vi "FUG_PowerSupply.SetOnOff.vi"(0 "i ref in":refnum<vi>, 2 "value":bool, 5 "error in (no error)":errorcluster, 7 "channelIndex":i32) -> (14 "i ref out":refnum<vi>, 19 "error out (no error)":errorcluster)   [LabVIEW 2014, in "FUG_PowerSupply.lvlib"]
doc: "This VI calculates the right current from the DB values, saves the actual set current to the I-Attribute and set´s the Set Current-Service."
uses:
  FUG_PowerSupply.lvlib
  CSCore/CSSystem/CoreDefs/CoreDefs.error_type.ctl
  CSCore/CSSystem/CoreDefs/CoreDefs.error_severity.ctl
  CSCore/CSApplicationBaseClasses/PSChannelBase/PSChannelBase.serviceType.ctl
  CSlibraries/UtilityLib/UtilityLib.valueStatus.ctl
  CSCore/CSApplicationBaseClasses/PSChannelBase/PSChannelBase.directionType.ctl
  CSlibraries-extern/DimLVEvent/LVDimInterface/LVDimInterface.lvlib
  CSCore/CSApplicationBaseClasses/PSChannelBase/PSChannelBase.lvlib
  CSlibraries/UtilityLib/UtilityLib.lvlib
  CSCore/CSSystem/CoreLib/CoreLib.lvlib
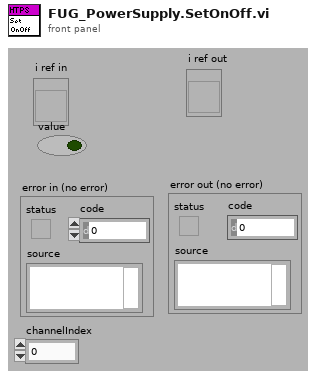
[diagram p1: front panel]
types:
  T1 = typedef "CoreDefs.error_severity.ctl" = enum16{"undefined", "information", "warning", "error", "fatal"}
  T2 = typedef "CoreDefs.error_type.ctl" = enum16{"no error", "can't load process", "can't unload process", "process does not exist", "can't install process", "can't remove process", "unknown function", "time out", "can't execute function", "duplicate queue name", "super not found", "caller queue invalid", "can't ping process", "unknown error", "VISA Error", "VISA timeout", "GPIB timeout", "GPIB error", "communication error", "data type mismatch", "can't read data from OPC server", "can't write data to OPC server", "OET error", "function not implemented", "process already exists", "invalid Shared Variable name", "error writing Shared Variable", "error reading Shared Variable", "invalid client name", "corrupt database", "unknown class", "call not authorized", "parameter out of range", "OET timeout: can't get data to modify", "invalid queue name", "requested operation incompatible with current state", "event undefined", "event disabled", "state undefined", "caller is not a friend", "EventBuilder: bad eventID", "EventBuilder: no DAQ devices", "a thread must not stop itself", "UNUSED ELEMENT4", "DiscArchiver: eventData incomplete", "DiscArchiver: eventData does not belong to run", "DiscArchiver: can't open file", "DiscArchiver: can't write to file", "DiscArchiver: available disc space low", "can't acquire semaphore", "error reading data from database", "notifier object is not existing", "can't register process", "can't unregister process", "illegal event type", "object disabled", "object already exists", "can't change state", "Instrument not found", "no connection to remote node", "invalid reference", "N/A", "UNUSED ELEMENT 1", "element not found", "illegal TCP/IP connection detected", "object does not exist", "invalid access ID", "unknown CS system", "invalid privilige", "unsupported data type", "unsupported server type", "IO server already exists", "Shared Variable already exists"}
  T3 = typedef "UtilityLib.lvlib/UtilityLib.valueStatus.ctl" = enum16{"no info available", "stand by/off", "on", "warning", "alarm/malfunction", "not implemented", "user action required", "important information", "system default", "control default", "indicator default", "button default"}
  T4 = typedef "PSChannelBase.lvlib/PSChannelBase.serviceType.ctl" = enum16{"onOff", "voltage", "current", "tripCurrent", "rampUpSpeed", "rampDownSpeed", "status"}
  T5 = typedef "PSChannelBase.lvlib/PSChannelBase.directionType.ctl" = enum16{"unknown", "update actual value", "update nominal value", "update both"}
  T6 = typedef "FUG_PowerSupply.lvlib/FUG_PowerSupply.i attribute.ctl" = cluster{"Type":string, "Elektrode Name":string, "CALC_FACTOR_SET_VOLTAGE":dbl, "CALC_FACTOR_GET_VOLTAGE":dbl, "CALC_FACTOR_GET_CURRENT":dbl, "CALC_FACTOR_SET_CURRENT ":dbl, "REG_VALUE":dbl, "Sign":bool, "setVoltID":i32, "setCurrentID":i32, "setPowerOnID":i32, "MaxVoltage":dbl}
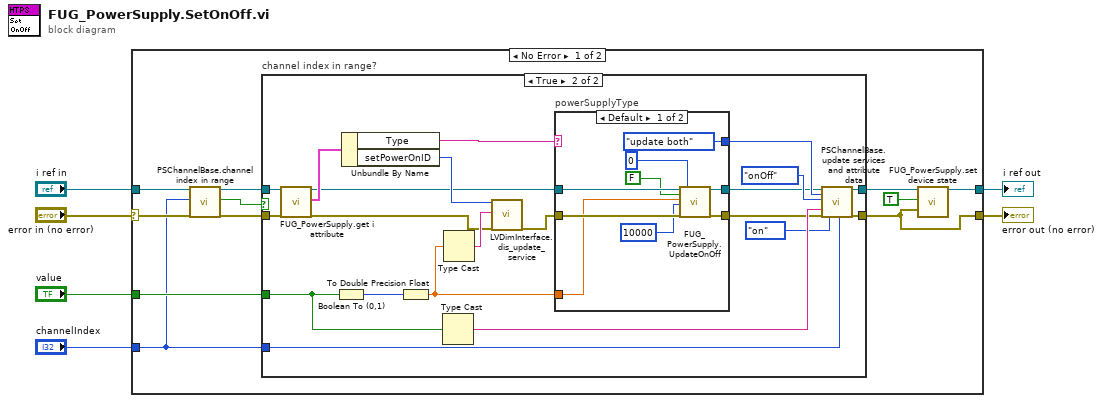
[diagram p0: block diagram]
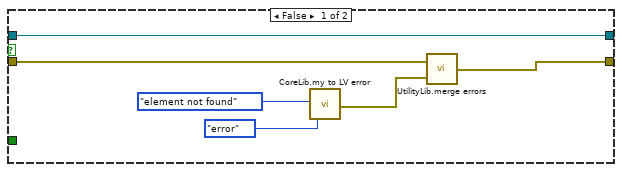
[diagram p2: hidden frame]
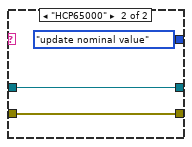
[diagram p3: hidden frame]
diagram:
  n1 = case shown="No Error" "error in (no error)" {
    selector: "error in (no error)" -> [w15 w58]
    tunnel: [w10 w58] -> w3
    tunnel: "i ref in" -> [w16 w57]
    tunnel: [w9 w57] -> w5
    tunnel: "value" -> [w17 _]
    tunnel: "channelIndex" -> [w7 _]
    frame No Error {
      n2 = call "PSChannelBase.channel index in range.vi"("i ref in"=w16, "channelIndex"=w7, "error in (no error)"=w15) -> ("i ref out"=w13:refnum<vi>, "in range"=w12:bool, "error out"=w14:errorcluster)  [unwired: 14 in]
      n3 = case "channel index in range?" shown="True" w12 {
        tunnel: w13 -> [w23 w41]
        tunnel: w14 -> [w20 w40]
        tunnel: w17 -> [_ w27]
        tunnel: [w18 w34] -> w10
        tunnel: [w23 w33] -> w11
        tunnel: w7 -> [_ w29]
        frame False {
          n4 = call "CoreLib.my to LV error.vi"("ErrorTypes"=CoreDefs.error_type."element not found", "severityLevel"=CoreDefs.error_severity."error") -> ("myErrorCluster"=w19:errorcluster)  [unwired: 16 in, 1 out]
          n5 = call "UtilityLib.merge errors.vi"("error2 (no error)"=w19, "error1 (no error)"=w20) -> ("error out"=w18:errorcluster)
        }
        frame True {
          n6 = call "FUG_PowerSupply.get i attribute.vi"("i ref in"=w41, "error in (no error)"=w40) -> ("i ref out"=w30:refnum<vi>, "i attribute"=w44:T6, "error out"=w39:errorcluster)  [unwired: 15 in]
          n7 = Boolean To (0,1)(Boolean=w27) -> (0, 1=w37:i16)
          n8 = Unbundle By Name(w44) -> ("Type"=w32:string, "setPowerOnID"=w43:i32)
          n9 = To Double Precision Float(number=w37) -> (double precision float=w24:dbl)
          n10 = Type Cast(x=w27) -> (*(type *) &x=w36:string)  [unwired: 1 in]
          n11 = Type Cast(x=w24) -> (*(type *) &x=w42:string)  [unwired: 1 in]
          n12 = call "LVDimInterface.dis_update_service.vi"("my_serviceID"=w43, "data"=w42, "error in (no error)"=w39) -> ("error out"=w28:errorcluster)  [unwired: 14 in, 2 out]
          n13 = case "powerSupplyType" shown="Default" w32 {
            tunnel: [PSChannelBase.directionType."update both" ("direction") PSChannelBase.directionType."update nominal value" ("direction")] -> w31
            tunnel: w30 -> [w52 w55]
            tunnel: w28 -> [w51 w54]
            tunnel: [w49 w55] -> w26
            tunnel: [w50 w54] -> w25
            tunnel: w24 -> [w48 _]
            frame Default {
              n14 = call "FUG_PowerSupply.UpdateOnOff.vi"("i ref in"=w52, "badValue"=FALSE, "moduleValue"=w48, "ms timeout (10000)"=10000, "error in (no error)"=w51, "onOffQuality"=0) -> ("i ref out"=w49:refnum<vi>, "error out"=w50:errorcluster)  [unwired: 11 in, 1 out]
            }
            frame "HCP65000" {
            }
          }
          n15 = call "PSChannelBase.update services and attribute data.vi"("i ref in"=w26, "direction"=w31, "service"=PSChannelBase.serviceType."onOff", "value"=w36, "error in (no error)"=w25, "quality"=UtilityLib.valueStatus."on", "channelNumber"=w29) -> ("i ref out"=w33:refnum<vi>, "error out"=w34:errorcluster)  [unwired: 10 in, 1 out]
        }
      }
      n16 = call "FUG_PowerSupply.set device state.vi"("i ref in"=w11, "implicit"=TRUE, "device error"=w10) -> ("i ref out"=w9:refnum<vi>)  [unwired: 14 in, 2 out]
    }
    frame Error {
    }
  }
  "error out (no error)" <- w3
  "i ref out" <- w5
